vi "readNameOfSelected.vi"(8 "error in (no error)":errorcluster, 11 "GoalUserInterface in":refnum<class "SingleSelectMCLBAdapter.lvclass">) -> (0 "error out":errorcluster, 2 "Name":string, 3 "GoalUserInterface out":refnum<class "SingleSelectMCLBAdapter.lvclass">)   [LabVIEW 2020, in "SingleSelectMCLBAdapter.lvclass"]
uses:
  SingleSelectMCLBAdapter.lvclass
  SingleSelectMCLBAdapter.lvclass/SingleSelectMCLBAdapter.ctl
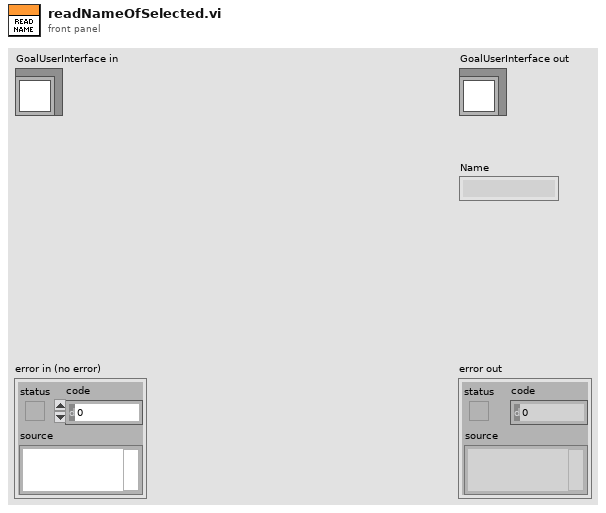
[diagram p1: front panel]
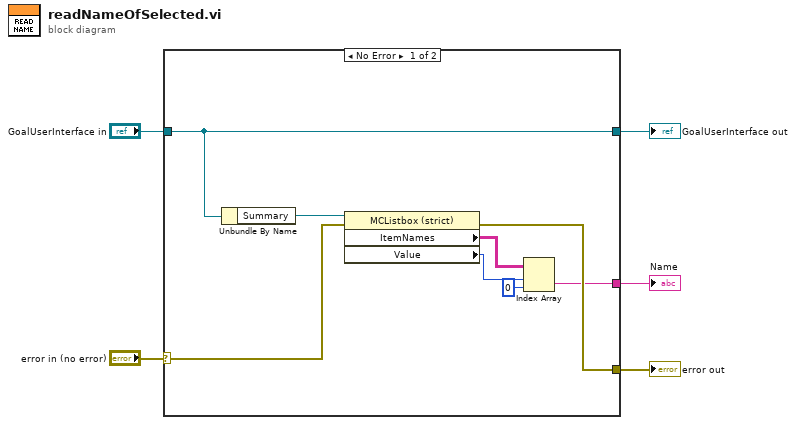
[diagram p0: block diagram]
diagram:
  n1 = case shown="No Error" "error in (no error)" {
    selector: "error in (no error)" -> [w12 w15]
    tunnel: [w8 w15] -> w4
    tunnel: [w9 w14] -> w2
    tunnel: "GoalUserInterface in" -> [w9 w14]
    tunnel: [w6 _] -> w1
    frame No Error {
      n2 = Unbundle By Name(w9) -> ("Summary"=w13:refnum<vi>)
      n3 = property class="MCListbox (strict)"(reference=w13, error in=w12) -> (error out=w8:errorcluster, "ItemNames"=w11:string[][], "Value"=w10:i32)  [unwired: 1 out]
      n4 = Index Array(array=w11, index (row)=w10, index (col)=0 ("disabled index (col)")) -> (element=w6:string)
    }
    frame Error {
    }
  }
  "error out" <- w4
  "GoalUserInterface out" <- w2
  "Name" <- w1
